vi "Msgbox - Add OR Remove.vi"(8 "Error In":errorcluster, 11 "MsgBox":T1={"Show"=TRUE, "Priority"=0, "Message"="", "seconds"=100}) -> (0 "Error Out":errorcluster, 3 "created new?":bool)   [LabVIEW 2013]
uses:
  Controls/Msgbox Timer Cluster.ctl
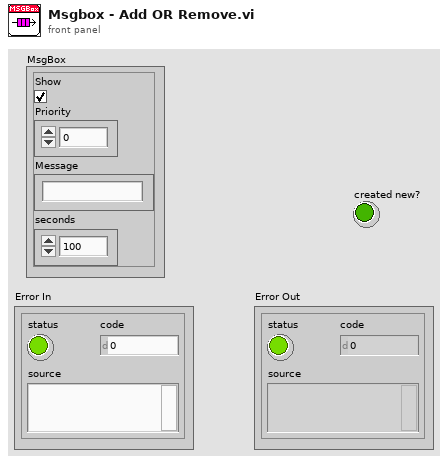
[diagram p1: front panel]
types:
  T1 = typedef "Msgbox Timer Cluster.ctl" = cluster{"Show":bool, "Priority":i32, "Message":string, "seconds":i32}
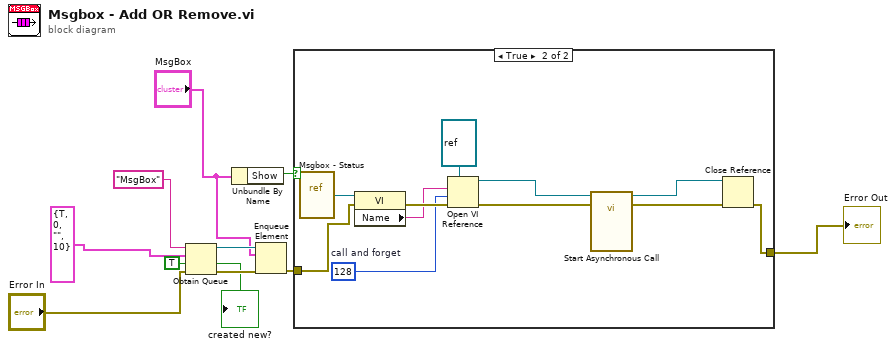
[diagram p0: block diagram]
diagram:
  n1 = Obtain Queue(name (unnamed)="MsgBox", element data type=T1 {"Show"=TRUE, "Priority"=0, "Message"="", "seconds"=10} ("MsgBox"), create if not found? (T)=TRUE, error in (no error)="Error In") -> (queue out=w7:refnum<queue>, created new?=→"created new?":bool, error out=w5:errorcluster)  [unwired: 1 in]
  n2 = Unbundle By Name("MsgBox") -> ("Show"=w8:bool)
  n3 = Enqueue Element(queue=w7, element="MsgBox", error in (no error)=w5) -> (error out=w3:errorcluster)  [unwired: 1 in, 2 out]
  n4 = case shown="True" w8 {
    tunnel: [w12 w14] -> w4
    tunnel: w3 -> [w12 w13]
    frame False {
    }
    frame True {
      w15 = 128  # call and forget
      n5 = vi-ref "Msgbox - Status.vi"() -> (w21:refnum<vi>)
      n6 = property class="VI"(reference=w21, error in=w13) -> (error out=w23:errorcluster, "Name"=w22:string)  [unwired: 1 out]
      n7 = Open VI Reference(type specifier VI Refnum (for type only)=refnum<vi> refnum, vi path=w22, options=w15, error in (no error)=w23) -> (vi reference=w17:refnum<vi>, error out=w18:errorcluster)  [unwired: 2 in]
      n8 = call-by-ref "Start Asynchronous Call"(reference=w17, error in=w18) -> (reference out=w20:refnum<vi>, error out=w19:errorcluster)  [unwired: 11 in, 1 out]
      n9 = Close Reference(reference=w20, error in (no error)=w19) -> (error out=w14:errorcluster)
    }
  }
  "Error Out" <- w4
